vi "Decode packages.vi"(11 "Array":bool[](array[boolean])) -> (1 "Value Out":u64, 2 "Version Sum":u64, 3 "Array Out":bool[](array[boolean]))   [LabVIEW 2021]
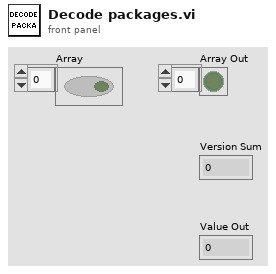
[diagram p1: front panel]
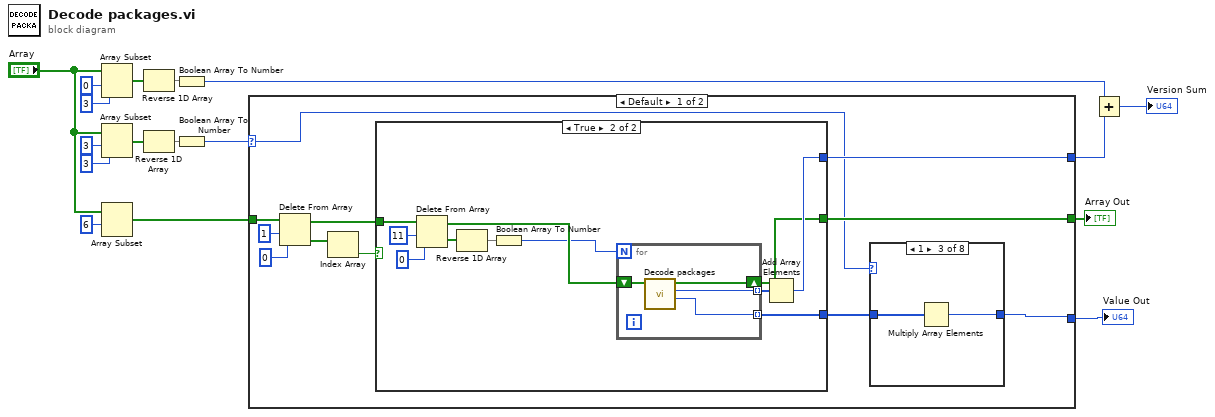
[diagram p0: block diagram]
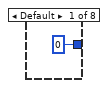
[diagram p2: hidden frame]
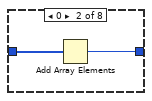
[diagram p3: hidden frame]
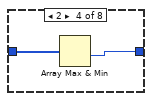
[diagram p4: hidden frame]
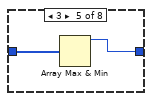
[diagram p5: hidden frame]
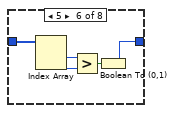
[diagram p6: hidden frame]
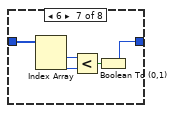
[diagram p7: hidden frame]
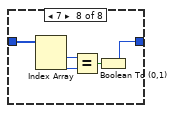
[diagram p8: hidden frame]
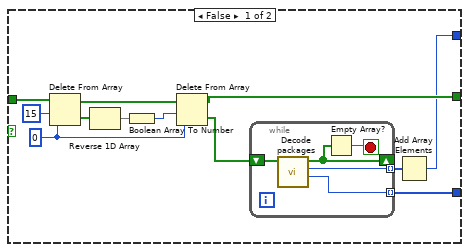
[diagram p9: hidden frame]
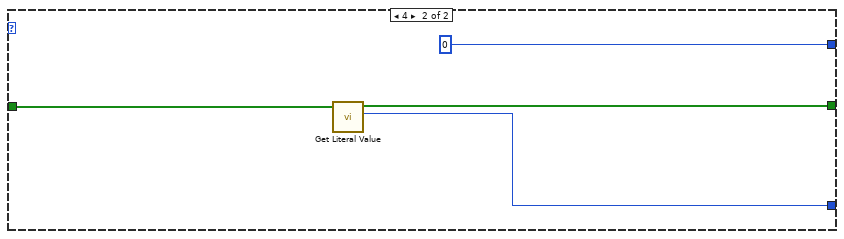
[diagram p10: hidden frame]
diagram:
  n1 = Array Subset(array="Array", index=0, length=3) -> (w7:bool[])
  n2 = Array Subset(array="Array", index=3, length=3) -> (w11:bool[])
  n3 = Array Subset(array="Array", index=6) -> (w14:bool[])  [unwired: 1 in]
  n4 = Reverse 1D Array(array=w7) -> (reversed array=w8:bool[])
  n5 = Reverse 1D Array(array=w11) -> (reversed array=w9:bool[])
  n6 = Boolean Array To Number(Boolean array=w8) -> (number=w15:u64)
  n7 = Boolean Array To Number(Boolean array=w9) -> (number=w10:u32)
  n8 = case shown="Default" w10 {
    selector: w10 -> [w20 _]
    tunnel: w14 -> [w27 w88]
    tunnel: [w18 w86] -> w2
    tunnel: [w21 u64 0 ("number")] -> w16
    tunnel: [w22 w85] -> w1
    frame Default {
      n9 = Delete From Array(array=w27, length=1, index=0) -> (deleted portion=w25:bool[], array with subset deleted=w26:bool[])
      n10 = Index Array(array=w25) -> (element=w28:bool)  [unwired: 1 in]
      n11 = case shown="True" w28 {
        tunnel: w26 -> [w63 w79]
        tunnel: [w57 w70] -> w22
        tunnel: [w54 w74] -> w21
        tunnel: [w53 w73] -> w19
        frame False {
          w58 = 0 ("index")
          n12 = Delete From Array(array=w63, length=15, index=w58) -> (deleted portion=w62:bool[], array with subset deleted=w60:bool[])
          n13 = Reverse 1D Array(array=w62) -> (reversed array=w61:bool[])
          n14 = Boolean Array To Number(Boolean array=w61) -> (number=w59:u32)
          n15 = Delete From Array(array=w60, length=w59, index=w58) -> (deleted portion=w56:bool[], array with subset deleted=w57:bool[])
          n16 = while {
            shift-right: [w67] -> _
            shift-left: w56 -> [w69]
            tunnel: [w68] -> w55 mode=indexing
            tunnel: [w65] -> w53 mode=indexing
            stop <- w66 stop-if-true
            n17 = call "Decode packages.vi"("Array"=w69) -> ("Value Out"=w65:u64, "Version Sum"=w68:u64, "Array Out"=w67:bool[])  [unwired: 8 in]
            n18 = Empty Array?(array=w67) -> (empty?=w66:bool)
          }
          n19 = Add Array Elements(numeric array=w55) -> (sum=w54:u64)
        }
        frame True {
          n20 = Delete From Array(array=w79, length=11, index=0) -> (deleted portion=w78:bool[], array with subset deleted=w72:bool[])
          n21 = Reverse 1D Array(array=w78) -> (reversed array=w77:bool[])
          n22 = Boolean Array To Number(Boolean array=w77) -> (number=w71:u32)
          n23 = for {
            N: w71 -> [_]
            shift-right: [w82] -> w70
            shift-left: w72 -> [w84]
            tunnel: [w83] -> w75 mode=indexing
            tunnel: [w81] -> w73 mode=indexing
            n24 = call "Decode packages.vi"("Array"=w84) -> ("Value Out"=w81:u64, "Version Sum"=w83:u64, "Array Out"=w82:bool[])  [unwired: 8 in]
          }
          n25 = Add Array Elements(numeric array=w75) -> (sum=w74:u64)
        }
      }
      n26 = case shown="1" w20 {
        tunnel: w19 -> [_ w31 w33 w35 w37 w42 w47 w52]
        tunnel: [u64 0 ("Value Out") w30 w32 w34 w36 w39 w44 w49] -> w18
        frame Default {
        }
        frame 0 {
          n27 = Add Array Elements(numeric array=w31) -> (sum=w30:u64)
        }
        frame 1 {
          n28 = Multiply Array Elements(1:w33) -> (0:w32:u64)
        }
        frame 2 {
          n29 = Array Max & Min(array=w35) -> (min value=w34:u64)  [unwired: 3 out]
        }
        frame 3 {
          n30 = Array Max & Min(array=w37) -> (max value=w36:u64)  [unwired: 3 out]
        }
        frame 5 {
          n31 = Index Array(array=w42) -> (element #1=w40:u64, element #2=w41:u64)  [unwired: 2 in]
          n32 = Greater?(x=w40, y=w41) -> (0:w38:bool)
          n33 = Boolean To (0,1)(Boolean=w38) -> (0, 1=w39:i16)
        }
        frame 6 {
          n34 = Index Array(array=w47) -> (element #1=w45:u64, element #2=w46:u64)  [unwired: 2 in]
          n35 = Less?(x=w45, y=w46) -> (x < y?=w43:bool)
          n36 = Boolean To (0,1)(Boolean=w43) -> (0, 1=w44:i16)
        }
        frame 7 {
          n37 = Index Array(array=w52) -> (element #1=w50:u64, element #2=w51:u64)  [unwired: 2 in]
          n38 = Equal?(x=w50, y=w51) -> (x = y?=w48:bool)
          n39 = Boolean To (0,1)(Boolean=w48) -> (0, 1=w49:i16)
        }
      }
    }
    frame 4 {
      n40 = call "Get Literal Value.vi"("Array In"=w88) -> ("Number"=w86:u64, "Array Out"=w85:bool[])  [unwired: 9 in]
    }
  }
  "Value Out" <- w2
  "Array Out" <- w1
  n41 = Add(x=w15, y=w16) -> (x+y=→"Version Sum":u64)
